vi "ComputeXYZ.vi"() -> ()   [LabVIEW 2011]
uses:
  <vilib>/vision/Image Controls.llb/IMAQ Image.ctl
panel:
  out "position":cluster{"X":sgl, "Y":sgl, "Z":sgl}
  in  "tracker":u64
  in  "Image":T1
  out "tracker":u64
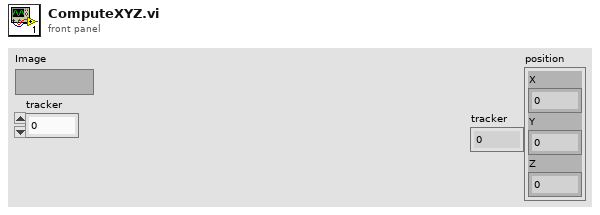
[diagram p1: front panel]
types:
  T1 = typedef "IMAQ Image.ctl" = refnum<image>
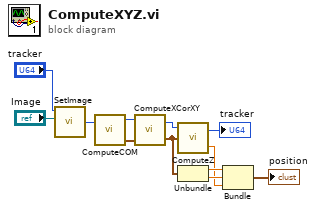
[diagram p0: block diagram]
diagram:
  n1 = call "SetImage.vi"("Image"="Image", "tracker"="tracker") -> ("tracker"=w3:u64)  [unwired: 2 in]
  n2 = call "ComputeCOM.vi"("tracker"=w3) -> ("tracker"=w2:u64, "position"=w1:cluster{"X":sgl, "Y":sgl})  [unwired: 1 in, 1 out]
  n3 = call "ComputeXCorXY.vi"("position"=w1, "tracker"=w2) -> ("position"=w8:cluster{"X":sgl, "Y":sgl}, "tracker"=w9:u64)  [unwired: 1 in]
  n4 = call "ComputeZ.vi"("position"=w8, "tracker"=w9) -> ("Z"=w5:sgl, "tracker"=→"tracker":u64)  [unwired: 1 in]
  n5 = Unbundle(w8) -> ("X"=w7:sgl, "Y"=w6:sgl)
  n6 = Bundle("X"=w7, "Y"=w6, "Z"=w5) -> (→"position":cluster{"X":sgl, "Y":sgl, "Z":sgl})  [unwired: 1 in]
